vi "Parse Tournament Data.vi"(11 "Tournament Data In":string) -> (3 "Tournament Data":T1)   [LabVIEW 2020]
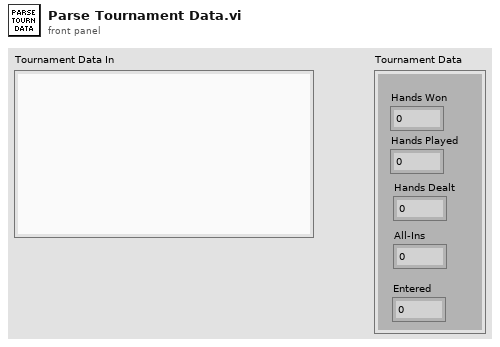
[diagram p1: front panel]
types:
  T1 = cluster{"Hands Won":i32, "Hands Played":i32, "Hands Dealt":i32, "All-Ins":i32, "Entered":dbl}
  T2 = cluster{"Stat Value":i32, "Stat Value":i32, "Stat Value":i32, "Stat Value":i32, "Stat Value":i32}
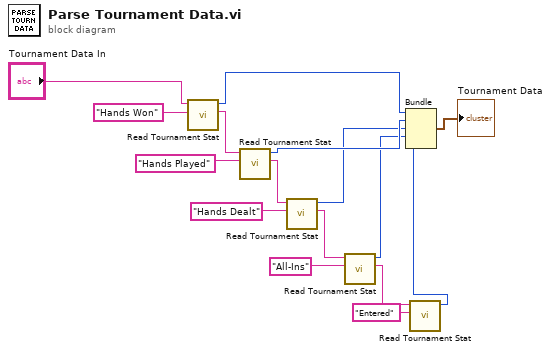
[diagram p0: block diagram]
diagram:
  n1 = call "Read Tournament Stat.vi"("Stat Name"="Hands Won" ("Stat String"), "Tournament Data In in"="Tournament Data In") -> ("Remaining String Out"=w14:string, "Stat Value"=w8:i32)  [unwired: 8 in]
  n2 = call "Read Tournament Stat.vi"("Stat Name"="Hands Played" ("regular expression"), "Tournament Data In in"=w14) -> ("Remaining String Out"=w13:string, "Stat Value"=w7:i32)  [unwired: 8 in]
  n3 = call "Read Tournament Stat.vi"("Stat Name"="Hands Dealt" ("regular expression"), "Tournament Data In in"=w13) -> ("Remaining String Out"=w12:string, "Stat Value"=w6:i32)  [unwired: 8 in]
  n4 = call "Read Tournament Stat.vi"("Stat Name"="All-Ins" ("regular expression"), "Tournament Data In in"=w12) -> ("Remaining String Out"=w3:string, "Stat Value"=w5:i32)  [unwired: 8 in]
  n5 = call "Read Tournament Stat.vi"("Stat Name"="Entered", "Tournament Data In in"=w3) -> ("Stat Value"=w1:i32)  [unwired: 8 in, 1 out]
  n6 = Bundle("Stat Value"=w8, "Stat Value"=w7, "Stat Value"=w6, "Stat Value"=w5, "Stat Value"=w1) -> (→"Tournament Data":T2)  [unwired: 1 in]
